vi "filterwheelcontrol_nothorlabslib.vi"(1 "Current OD filt":u16(ring)=1 caption="Current laser OD value" items=["OD 0"=1, "OD 0.5"=2, "OD 1"=3, "OD 2"=4, "OD 3"=5, "OD 4"=6], 2 "New ODfilt":u16(ring)=1 caption="New IR laser OD value" items=["OD 0"=1, "OD 0.5"=2, "OD 1"=3, "OD 2"=4, "OD 3"=5, "OD 4"=6]) -> ()   [LabVIEW 2015]
uses:
  <vilib>/DAQmx/write.llb/DAQmx Write (Digital Wfm 1Chan NSamp).vi
  <vilib>/Waveform/DWDTOps.llb/DWDT Analog to Digital.vi
  <vilib>/DAQmx/create/channels.llb/DAQmx Create Channel (DO-Digital Output).vi
  <vilib>/DAQmx/configure/timing.llb/DAQmx Timing (Sample Clock).vi
  <vilib>/Waveform/DWDTOps.llb/DWDT Uncompress Digital.vi
  <vilib>/DAQmx/miscellaneous.llb/DAQmx Fill In Error Info.vi
  <vilib>/measure/NI_MABase.lvlib
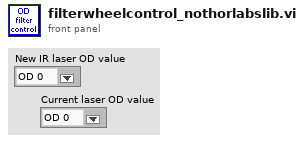
[diagram p1: front panel]
types:
  T1 = cluster{"StageS":i32, "StageL":i32, "currmeas data dir":path, "image OD":u16, "contour OD":u16, "point OD":u16, "AOlines":tag[], "AIlines":tag[], "CI lines":tag[], "DO lines":tag[], "AO names":string[], "CI names":string[], "AI names":string[], "DO names":string[], "CIextensions":string[], "AIextensions":string[], "Voltage to Ygalvo":i32, "Voltage to Xgalvo":i32, "Voltage to patch":i32, "640 shutter":i32, "2P shutter":i32, "LT timestamp":u32, "Vp":i32, "Ip":i32, "camera trigger":i32, "master data dir":path, "voltage to Zpos":i32, "Vto2P":i32, "640 AO":i32, "488 AO":i32, "532 AO":i32, "640TTL":u32, "488TTL":u32, "532TTL":u32, "Device 1 sampleclock out":tag, "Device 1 Starttrigger out":tag, "Device 2 sampleclock in":tag, "Device 2 StartTrigger in ":tag, "2PODTTL":u32, "488 shutter":u32, "LCVR red":u32, "LCVR blue":u32}
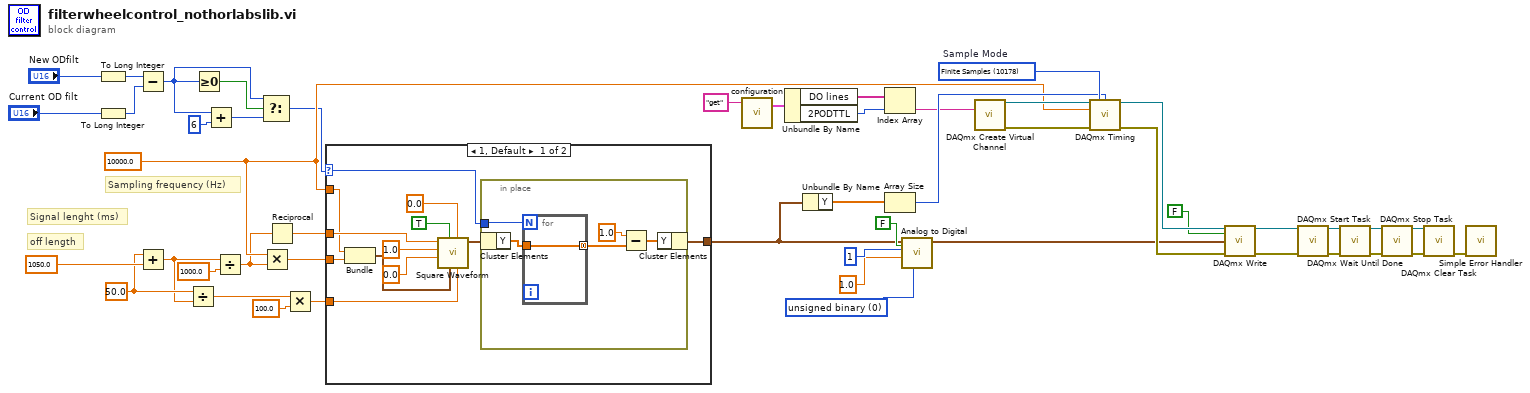
[diagram p0: block diagram]
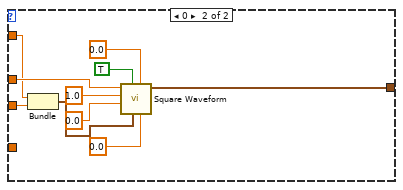
[diagram p2: hidden frame]
diagram:
  w15 = 50.0 ("length of command (ms)")
  w28 = 10000.0 ("element")
  w36 = u16 0 items=["unsigned binary", "offset binary", "2's complement"] ("data format (offset binary)")
  w42 = 10178 items=["Finite Samples"=10178, "Continuous Samples"=10123, "Hardware Timed Single Point"=12522]  # Sample Mode
  # "off length"
  # "Signal lenght (ms)"
  # "Sampling frequency (Hz)"
  n1 = To Long Integer(number="New ODfilt") -> (32bit integer=w21:i32)
  n2 = To Long Integer(number="Current OD filt") -> (32bit integer=w20:i32)
  n3 = Subtract(x=w21, y=w20) -> (x-y=w24:i32)
  n4 = Add(x=w15, y=1050.0 ("length of command (ms)")) -> (x+y=w14:dbl)
  n5 = Divide(x=w15, y=w14) -> (x/y=w13:dbl)
  n6 = Greater Or Equal To 0?(x=w24) -> (x >= 0?=w25:bool)
  n7 = Add(x=w24, y=6) -> (x+y=w22:i32)
  n8 = Divide(x=w14, y=1000.0) -> (x/y=w18:dbl)
  n9 = Select(t=w24, s=w25, f=w22) -> (s? t:f=w7:i32)
  n10 = Multiply(x=w28, y=w18) -> (x*y=w27:dbl)
  n11 = Reciprocal(x=w18) -> (1/x=w17:dbl)
  n12 = Multiply(x=w13, y=100.0) -> (x*y=w10:dbl)
  n13 = case shown="1, Default" w7 {
    selector: w7 -> [w51 _]
    tunnel: w27 -> [w59 w68]
    tunnel: w17 -> [w56 w73]
    tunnel: w28 -> [w53 w70]
    tunnel: [w50 w69] -> w11
    tunnel: w10 -> [w49 _]
    frame 1, Default {
      n14 = Bundle("element"=w53, w59) -> (w60:cluster{"element":dbl, dbl})  [unwired: 1 in]
      n15 = call <vilib>:"Square Waveform.vi"("duty cycle (%)"=w49, "offset"=0.0, "sampling info"=w60, "reset signal"=TRUE, "phase"=0.0, "amplitude"=1.0, "frequency"=w56) -> ("signal out"=w52:waveform(dbl))  [unwired: 3 in, 1 out]
      n16 = in-place {
        in-place-border: w51 -> [w65]
        n17 = in-place-cluster #1(w52) -> ("Y"=w64:dbl[])
        n18 = for {
          N: w65 -> [_]
          tunnel: w64 -> [w66]
          tunnel: [w66] -> w63 mode=concatenating
        }
        n19 = Subtract(x=1.0, y=w63) -> (x-y=w62:dbl[])
        n20 = in-place-cluster #1("Y"=w62) -> (w50:waveform(dbl))
      }
    }
    frame 0 {
      n21 = Bundle("element"=w70, w68) -> (w76:cluster{"element":dbl, dbl})  [unwired: 1 in]
      n22 = call <vilib>:"Square Waveform.vi"("duty cycle (%)"=0.0, "offset"=0.0, "sampling info"=w76, "reset signal"=TRUE, "phase"=0.0, "amplitude"=1.0, "frequency"=w73) -> ("signal out"=w69:waveform(dbl))  [unwired: 3 in, 1 out]
    }
  }
  n23 = call "configuration.vi"("command"="get") -> ("config out"=w4:T1)  [unwired: 2 in, 1 out]
  n24 = Unbundle By Name(w4) -> ("DO lines"=w3:tag[], "2PODTTL"=w2:u32)
  n25 = Unbundle By Name(w11) -> ("Y"=w12:dbl[])
  n26 = Index Array(array=w3, index=w2) -> (element=w1:tag)
  n27 = Array Size(array=w12) -> (size(s)=w30:i32)
  n28 = call-poly <vilib>:"Analog to Digital.vi"("data format (offset binary)"=w36, "compress digital (T)"=FALSE, "full-scale range (pk-pk)"=1.0, "resolution (16 bit)"=1, "analog waveform"=w11) -> ("digital waveform"=w8:digitalwaveform)  [unwired: 3 in, 3 out]
  n29 = call-poly <vilib>:"DAQmx Create Virtual Channel.vi"("lines"=w1) -> ("task out"=w40:refnum<k21>, "error out"=w41:errorcluster)  [unwired: 13 in]
  n30 = call-poly <vilib>:"DAQmx Timing.vi"("task/channels in"=w40, "sample mode"=w42, "samples per channel"=w30, "rate"=w28, "error in"=w41) -> ("task out"=w47:refnum<k21>, "error out"=w48:errorcluster)  [unwired: 9 in]
  n31 = call-poly <vilib>:"DAQmx Write.vi"("task/channels in"=w47, "auto start"=FALSE, "data"=w8, "error in"=w48) -> ("task out"=w45:refnum<k21>, "error out"=w46:errorcluster)  [unwired: 9 in, 1 out]
  n32 = call <vilib>:"DAQmx Start Task.vi"("task/channels in"=w45, "error in"=w46) -> ("task out"=w34:refnum<k21>, "error out"=w32:errorcluster)  [unwired: 12 in]
  n33 = call <vilib>:"DAQmx Wait Until Done.vi"("task/channels in"=w34, "error in"=w32) -> ("task out"=w33:refnum<k21>, "error out"=w31:errorcluster)  [unwired: 12 in]
  n34 = call <vilib>:"DAQmx Stop Task.vi"("task/channels in"=w33, "error in"=w31) -> ("task out"=w44:refnum<k21>, "error out"=w43:errorcluster)  [unwired: 12 in]
  n35 = call <vilib>:"DAQmx Clear Task.vi"("task in"=w44, "error in"=w43) -> ("error out"=w39:errorcluster)  [unwired: 13 in]
  n36 = call <vilib>:"Simple Error Handler.vi"("error in (no error)"=w39) -> ()  [unwired: 4 in, 5 out]
